vi "acq.Filename.vi"(9 "module":string) -> (1 "filename":string)   [LabVIEW 2020]
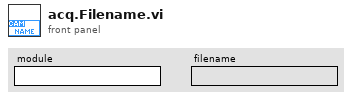
[diagram p1: front panel]
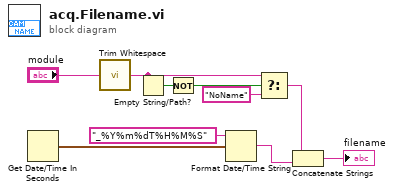
[diagram p0: block diagram]
diagram:
  n1 = Get Date/Time In Seconds() -> (seconds since 1Jan1904=w9:timestamp)
  n2 = call <vilib>:"Trim Whitespace.vi"("string"="module") -> ("trimmed string"=w4:string)  [unwired: 1 in]
  n3 = Empty String/Path?(string/path=w4) -> (empty?=w5:bool)
  n4 = Not(x=w5) -> (.not. x?=w3:bool)
  n5 = Format Date/Time String(time format string (%c)="_%Y%m%dT%H%M%S", seconds (now)=w9) -> (date/time string=w7:string)  [unwired: 1 in]
  n6 = Select(t=w4, s=w3, f="NoName") -> (s? t:f=w2:string)
  n7 = Concatenate Strings(w2, w7) -> (→"filename":string)
